vi "LVClass_WavefrontCorrectorSet Get Parameter Option.vi"(0 "WavefrontCorrectorSet in":refnum<class "WavefrontCorrectorSet.lvclass">, 5 "parameter_name":string, 11 "error in (no error)":errorcluster) -> (3 "Settable-Gettable?":cluster{"Settable":bool, "Gettable":bool}, 4 "WavefrontCorrectorSet out":refnum<class "WavefrontCorrectorSet.lvclass">, 6 "DefaultValueExist":bool, 8 "minmax":bool, 10 "String enum":bool, 13 "is_connection_parameter?":bool, 14 "Settable-Gettable on fly?":cluster{"Settable":bool, "Gettable":bool}, 15 "error out":errorcluster)   [LabVIEW 2020, in "WavefrontCorrectorSet.lvclass"]
doc: "WavefrontCorrector parameter options getter given its name which should have\nbeen read with Imop_WavefrontCorrectorSet_GetParameterName.\n\n--------------------------------------------------------------------------------\n\n<B>wavefrontcorrector_setIn </B> : WavefrontCorrectorSet object.\n<B>wavefrontcorrector_setOut </B> : WavefrontCorrectorSet object.\n<B>parameter_name </B> : Parameter name.\n<B>is_settable </B> : Parameter value is writeable.\n<B>is_gettable </B> : Parameter value is readable.\n<B>has_default_value </B> : Parameter has a default value.\n<B>has_limits </B> : If parameter is a number, its value is to be selected between a min and a max\n value.\n<B>is_string_enum </B> : If parameter is a string, its value is to be selected in a finite set of\n values.\n<B>is_settable_on_fly </B> : Parameter is writeable while wavefront corrector is running, and a value\n change is taken into account asap.\n<B>is_gettable_on_fly </B> : Parameter is readable while wavefront correcto is running, and the return\n value will be the one currently used.\n<B>ErrorIn </B> : Error\n<B>ErrorOut </B> : Error\n\n--------------------------------------------------------------------------------"
uses:
  WavefrontCorrectorSet.lvclass
  WavefrontCorrectorSet.lvclass/WavefrontCorrectorSet.ctl
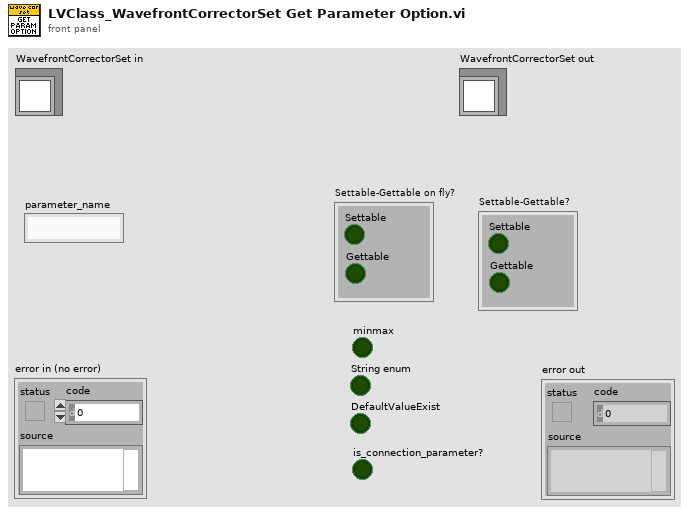
[diagram p1: front panel]
types:
  T1 = typedef "ClassID.ctl" = i64
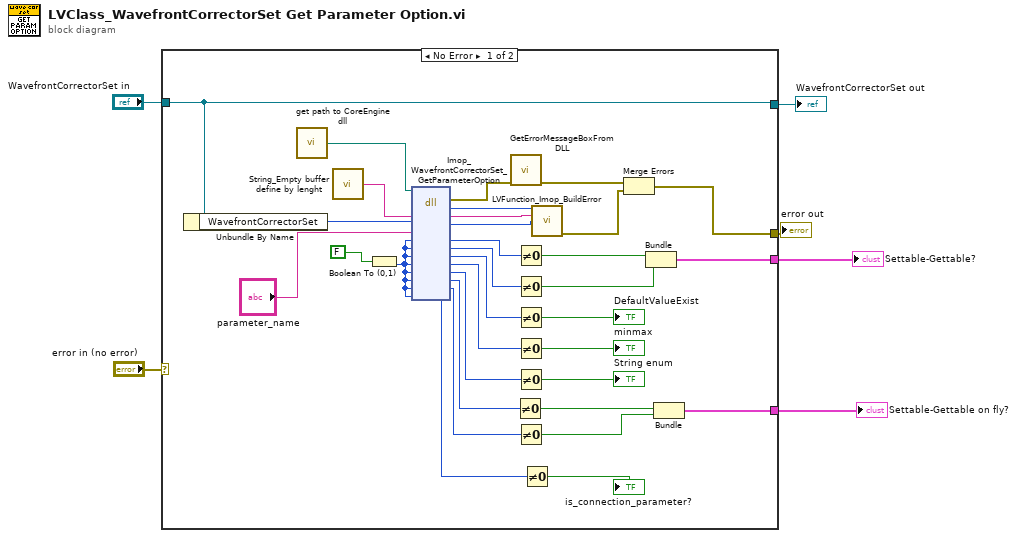
[diagram p0: block diagram]
diagram:
  n1 = case shown="No Error" "error in (no error)" {
    selector: "error in (no error)" -> [_ w39]
    tunnel: "WavefrontCorrectorSet in" -> [w23 w40]
    tunnel: [w23 w40] -> w3
    tunnel: [w19 w39] -> w4
    tunnel: [w17 _] -> w6
    tunnel: [w11 _] -> w5
    frame No Error {
      n2 = Unbundle By Name(w23) -> ("WavefrontCorrectorSet"=w22:T1)
      n3 = call "get path to CoreEngine dll.vi"() -> ("path to wavekit library"=w34:path)  [unwired: 14 in, 1 out]
      n4 = call "String_Empty buffer define by lenght.vi"() -> ("Empty buffer"=w36:string)  [unwired: 1 in]
      n5 = Boolean To (0,1)(Boolean=FALSE) -> (0, 1=w10:i16)
      n6 = dll-call lib="D:/soft/HASO_v3/C_interface/Sources/Build/vc100/Release/c_interface_vc100.dll" fn="Imop_WavefrontCorrectorSet_GetParameterOption"(path in=w34, "message"=w36, "objet"=w22, "parameter_name"="parameter_name", "Settable"=w10, "Gettable"=w10, "DefaultValueExist"=w10, "minmax"=w10, "StringEnum"=w10, "Settable_onfly"=w10, "Gettable_onfly"=w10, "is_connection_parameter"=w10) -> (error out=w33:errorcluster, "return type"=w38:i32, "message"=w37:string, "objet"=w7:i64, "Settable"=w31:u8, "Gettable"=w30:u8, "DefaultValueExist"=w29:u8, "minmax"=w27:u8, "StringEnum"=w25:u8, "Settable_onfly"=w15:u8, "Gettable_onfly"=w14:u8, "is_connection_parameter"=w9:u8)  [unwired: 3 in, 1 out]
      n7 = call "GetErrorMessageBoxFromDLL.vi"("error IN"=w33) -> ("error OUT"=w21:errorcluster)  [unwired: 10 in]
      n8 = Not Equal To 0?(x=w15) -> (x != 0?=w13:bool)
      n9 = Not Equal To 0?(x=w31) -> (x != 0?=w18:bool)
      n10 = Not Equal To 0?(x=w30) -> (x != 0?=w16:bool)
      n11 = Not Equal To 0?(x=w29) -> (x != 0?=→"DefaultValueExist":bool)
      n12 = Not Equal To 0?(x=w27) -> (x != 0?=→"minmax":bool)
      n13 = Not Equal To 0?(x=w25) -> (x != 0?=→"String enum":bool)
      n14 = Not Equal To 0?(x=w14) -> (x != 0?=w12:bool)
      n15 = Not Equal To 0?(x=w9) -> (x != 0?=→"is_connection_parameter?":bool)
      n16 = call "LVFunction_Imop_BuildError.vi"("code"=w38, "String to Prepend to source (\"\")"=w37, "Adresse"=w7) -> ("error out"=w20:errorcluster)  [unwired: 12 in]
      n17 = Merge Errors(w21, w20) -> (w19:errorcluster)
      n18 = Bundle(w18, w16) -> (w17:cluster{bool, bool})  [unwired: 1 in]
      n19 = Bundle(w13, w12) -> (w11:cluster{bool, bool})  [unwired: 1 in]
    }
    frame Error {
    }
  }
  "error out" <- w4
  "WavefrontCorrectorSet out" <- w3
  "Settable-Gettable?" <- w6
  "Settable-Gettable on fly?" <- w5
